vi "XIPIN_Reed-Solomon_Decoder_9_0.vi"   [LabVIEW 2017]
doc: "The Xilinx Reed-Solomon Decoder LogiCORE is a high speed, compact module that can be configured to implement many different Reed-Solomon coding standards. The core is fully synchronous, using a single clock, and supports continuous input data with no gap between code blocks. The core is parameterizable, allowing designers to control the symbol size, the code block length, the number of errors corrected, and the control signal behavior. The Decoder supports both error and erasure decoding. It is delivered through the Vivado IP Catalog and integrates seamlessly with the Xilinx design flow.\n------------------------------------\n<b>Need License</b> : Yes\n<b>Interface</b> : AXI4-Stream"
uses:
  <vilib>/rvi/XilinxIP/XIPIN_XNode/niFpgaXIPIN.xnode
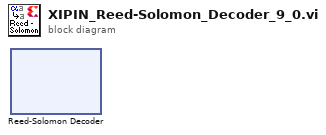
[diagram p0: block diagram]
diagram:
  n1 = xnode ("Reed-Solomon Decoder")() -> ()
